vi "WinTaskbar.vi"(8 "error in (no error)":errorcluster, 11 "Hide":bool) -> (0 "error out":errorcluster)   [LabVIEW 2020, in "WinAPI.lvlib"]
uses:
  WinAPI.lvlib
  C:/Users/dzoni/Documents/NJ/Playground/LV/WinAPI/DLL/WinAPI.dll
  DLL/WinAPI.dll
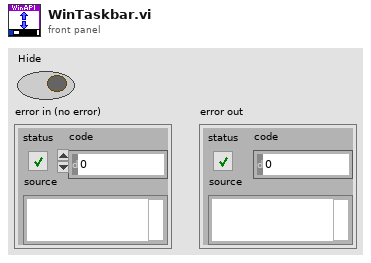
[diagram p1: front panel]
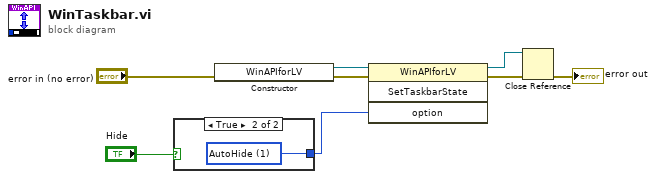
[diagram p0: block diagram]
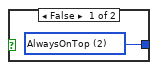
[diagram p2: hidden frame]
diagram:
  n1 = case shown="True" "Hide" {
    tunnel: [w9 w10] -> w5
    frame False {
      w9 = 2 items=["AutoHide"=1, "AlwaysOnTop"=2] ("option")
    }
    frame True {
      w10 = 1 items=["AutoHide"=1, "AlwaysOnTop"=2] ("option")
    }
  }
  n2 = constructor class="WinAPIforLV"(error in="error in (no error)") -> (reference out=w4:refnum<k24>, error out=w3:errorcluster)  [unwired: 2 in, 1 out]
  n3 = invoke class="WinAPIforLV" method="SetTaskbarState"(reference=w4, error in=w3, "option"=w5) -> (reference out=w7:refnum<k24>, error out=w6:errorcluster)  [unwired: 1 in, 2 out]
  n4 = Close Reference(reference=w7, error in (no error)=w6) -> (error out=→"error out":errorcluster)
